vi "G# - Polymorphism demo.vi"() -> ()   [LabVIEW 2020]
doc: "Polymorphism\nThis demo will show polymorphism in action.\n\nFour objects are created from different classes in a hierarchy. All objects references are casted to a DemoClass1 reference type. The virtual dynamic dispatch method \"MyMethod1\" will be executed for each of the objects and correct implementation will be used depending on the reference run time type.\n\nBy using the G# Debugger found in Tools->G# Debugger a text log can be followed showing how the objects were created and destroyed."
uses:
  DemoClass1_class/DemoClass1.lvclass
  DemoSubClass1_class/DemoSubClass1.lvclass
  C:/ProjectGSharpDevelopment_2020-3/gsharp/VIPM/Files/examples/Object-Oriented G# Development/Polymorphism/DemoClass1_class/DemoClass1.lvclass
  DemoSubSubClass1_class/DemoSubSubClass1.lvclass
  DemoSubClass2_class/DemoSubClass2.lvclass
  vi.lib/addons/_AddQ/G#Object/G#Object.lvclass
panel:
  in  "error in (no error)":errorcluster
  out "error out":errorcluster
  # "Polymorphism\nThis demo will show polymorphism in action.\n\nFour objects are created from different classes in a hierarchy. All objects references are casted to a DemoClass1 reference type.\nThe virtual dynamic dispatch method \"MyMethod1\" will be executed for each of the objects and correct implementation will be used depending on the reference run time type.\n\nBy using the G# Debugger found in Tools->G# Debugger a text log can be followed showing how the objects were created and destroyed."
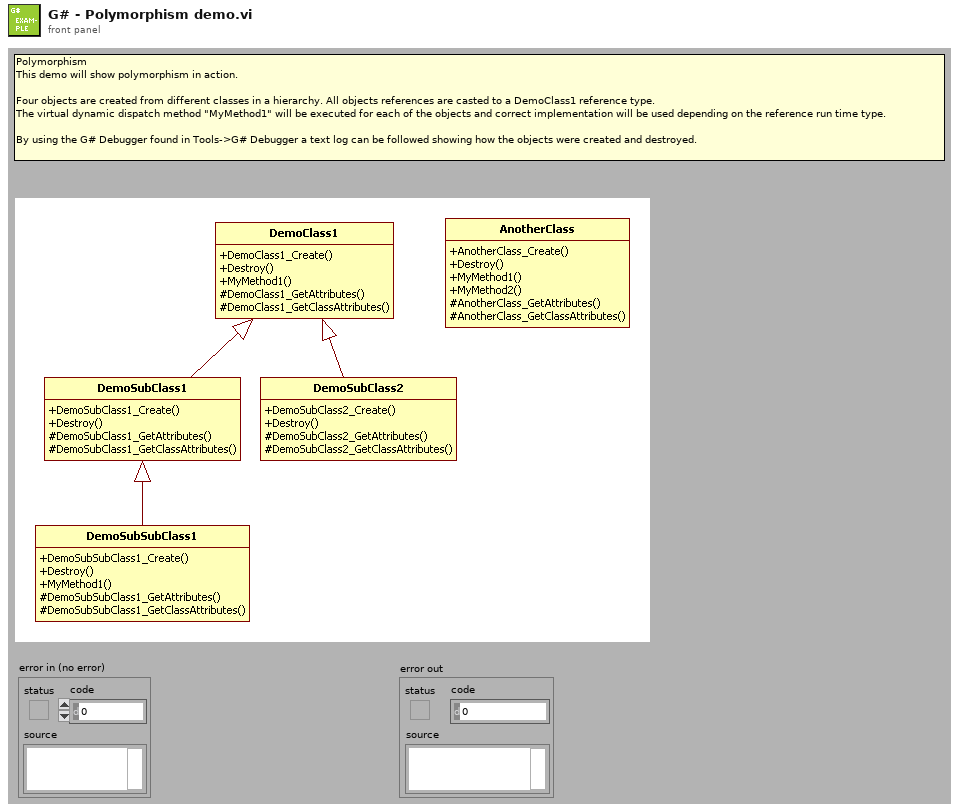
[diagram p1: front panel]
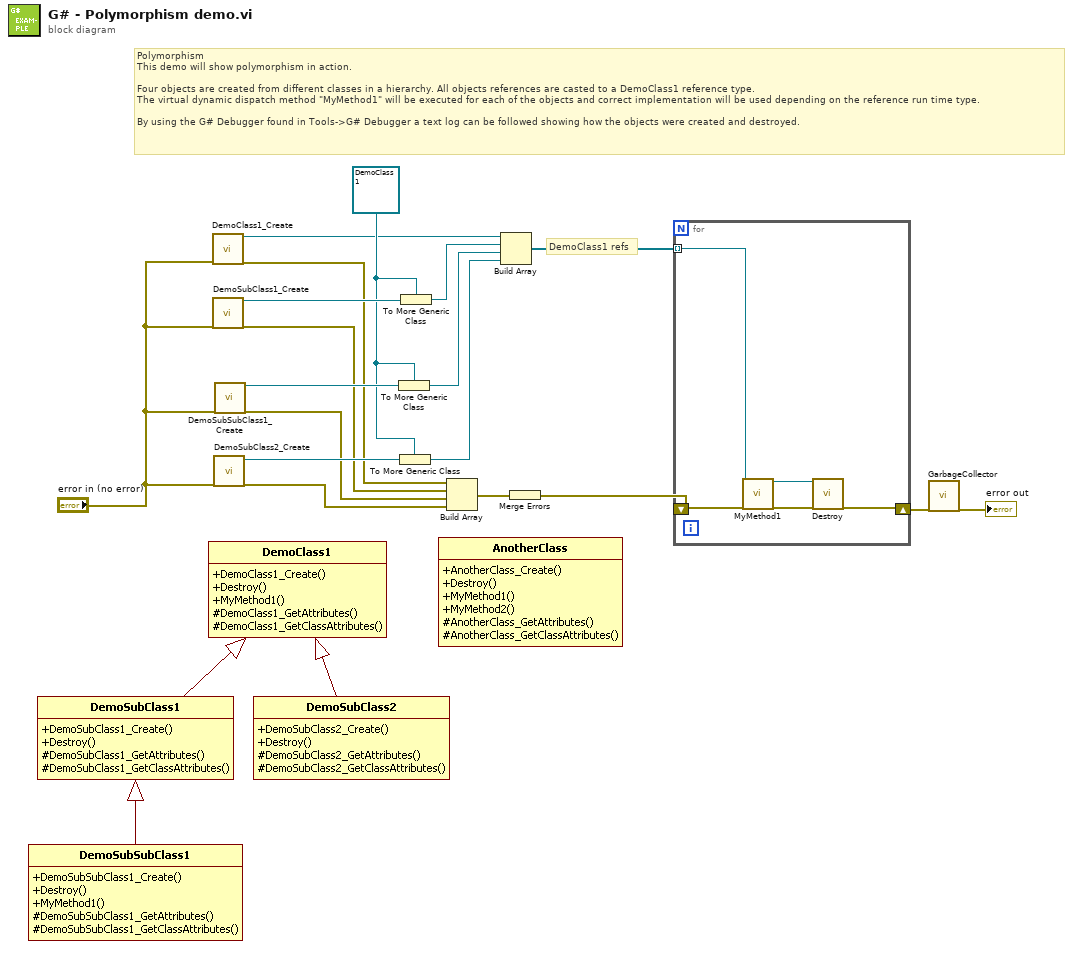
[diagram p0: block diagram]
diagram:
  w16 = refnum<class "DemoClass1.lvclass"> refnum ("DemoClass1.lvclass")
  # "Polymorphism\nThis demo will show polymorphism in action.\n\nFour objects are created from different classes in a hierarchy. All objects references are casted to a DemoClass1 reference type.\nThe virtual dynamic dispatch method \"MyMethod1\" will be executed for each of the objects and correct implementation will be used depending on the reference run time type.\n\nBy using the G# Debugger found in Tools->G# Debugger a text log can be followed showing how the objects were created and destroyed."
  # "DemoClass1 refs"
  n1 = call "DemoClass1_Create.vi"("error in (no error)"="error in (no error)") -> ("reference out"=w14:refnum<class "DemoClass1.lvclass">, "error out"=w10:errorcluster)  [unwired: 17 out]
  n2 = call "DemoSubClass1_Create.vi"("error in (no error)"="error in (no error)") -> ("reference out"=w18:refnum<class "DemoSubClass1.lvclass">, "error out"=w9:errorcluster)  [unwired: 17 out]
  n3 = call "DemoSubClass2_Create.vi"("error in (no error)"="error in (no error)") -> ("reference out"=w15:refnum<class "DemoSubClass2.lvclass">, "error out"=w7:errorcluster)  [unwired: 17 out]
  n4 = call "DemoSubSubClass1_Create.vi"("error in (no error)"="error in (no error)") -> ("reference out"=w17:refnum<class "DemoSubSubClass1.lvclass">, "error out"=w8:errorcluster)  [unwired: 17 out]
  n5 = To More Generic Class(target class=w16, reference=w17) -> (generic class reference=w12:refnum<class "DemoClass1.lvclass">)
  n6 = To More Generic Class(target class=w16, reference=w15) -> (generic class reference=w11:refnum<class "DemoClass1.lvclass">)
  n7 = To More Generic Class(target class=w16, reference=w18) -> (generic class reference=w13:refnum<class "DemoClass1.lvclass">)
  n8 = Build Array(w10, w9, w8, w7) -> (w6:errorcluster[])
  n9 = Build Array(w14, w13, w12, w11) -> (w5:refnum<class "DemoClass1.lvclass">[])
  n10 = Merge Errors(w6) -> (w4:errorcluster)
  n11 = for {
    tunnel: w5 -> [w22] mode=indexing
    shift-right: [w20] -> w3
    shift-left: w4 -> [w23]
    n12 = call-dynamic "MyMethod1.vi"("reference in"=w22, "error in (no error)"=w23) -> ("reference out"=w19:refnum<class "DemoClass1.lvclass">, "error out"=w21:errorcluster)  [unwired: 16 out]
    n13 = call-dynamic "Destroy.vi"("reference in"=w19, "error in (no error)"=w21) -> ("error out"=w20:errorcluster)  [unwired: 17 out]
  }
  n14 = call "GarbageCollector.vi"("error in (no error)"=w3) -> ("error out"=→"error out":errorcluster)  [unwired: 16 in, 2 out]
